vi "Get Serial Number.vi"(8 "error in (no error)":errorcluster, 11 "Barcode Reader in":refnum<class "Barcode Reader.lvclass">) -> (0 "error out":errorcluster, 2 "Serial Number":string, 3 "Barcode Reader out":refnum<class "Barcode Reader.lvclass">)   [LabVIEW 2020, in "Barcode Reader First Iteration.lvlib" / "Barcode Reader.lvclass"]
uses:
  Barcode Reader.lvclass
  Barcode Reader.lvclass/Barcode Reader.ctl
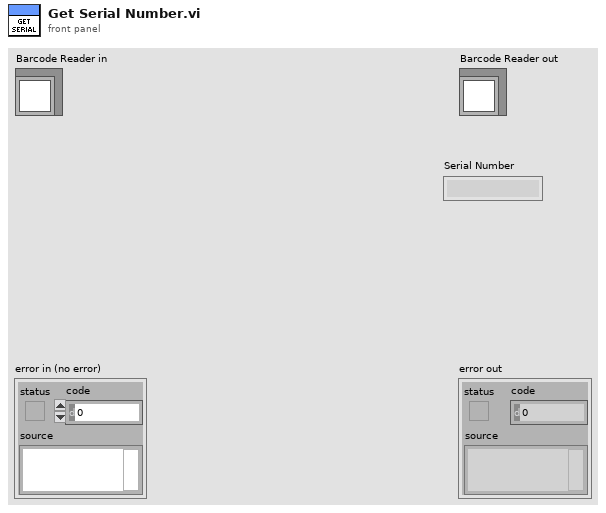
[diagram p1: front panel]
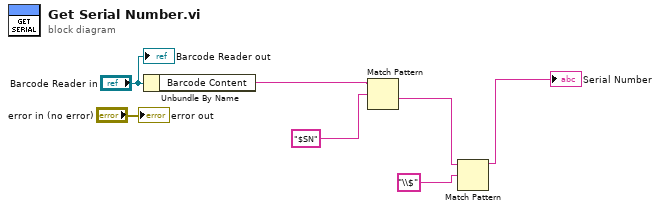
[diagram p0: block diagram]
diagram:
  n1 = Unbundle By Name("Barcode Reader in") -> ("Barcode Content"=w5:string)
  n2 = Match Pattern(string=w5, regular expression="$SN" ("format string")) -> (after substring=w3:string)  [unwired: 1 in, 3 out]
  n3 = Match Pattern(string=w3, regular expression="\\$" ("format string")) -> (before substring=→"Serial Number":string)  [unwired: 1 in, 3 out]
  "error out" <- "error in (no error)"
  "Barcode Reader out" <- "Barcode Reader in"
